vi "Keithley 2450 Read Multiple.vi"() -> ()   [LabVIEW 2024]
doc: "This example shows how to configure a measurement and take multiple readings."
uses:
  C:/Users/Public/OneDrive/Desktop/Keithley_2450_2470_1_4_0_LV2015_NewReadme2_2450-LV2015-1.4.0/Keithley 2450/Keithley 2450.lvlib
panel:
  in  "Compliance Level (0.1)":dbl=0.1
  in  "Output Level (0)":dbl
  in  "Source Mode  (0: Voltage)":u16(ring) items=["Voltage", "Current"]
  out "Resistance":sgl[](array[numeric])
  out "Current":sgl[](array[numeric])
  out "Voltage":sgl[](array[numeric])
  in  "VISA resource name":refnum<visa-resource-name>
  # "(c) 2021 National Instruments.  ALL RIGHTS RESERVED."
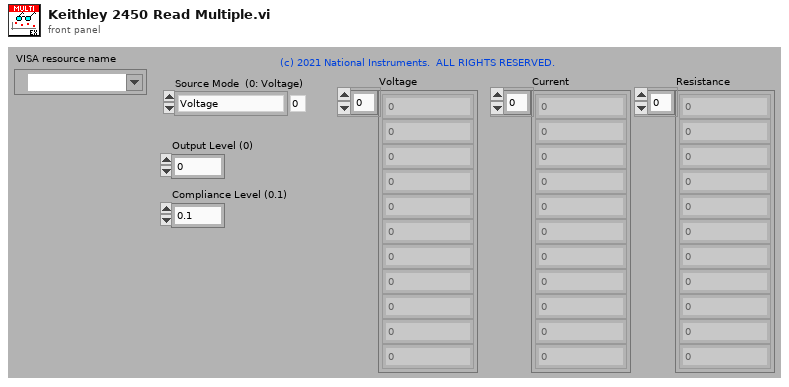
[diagram p1: front panel]
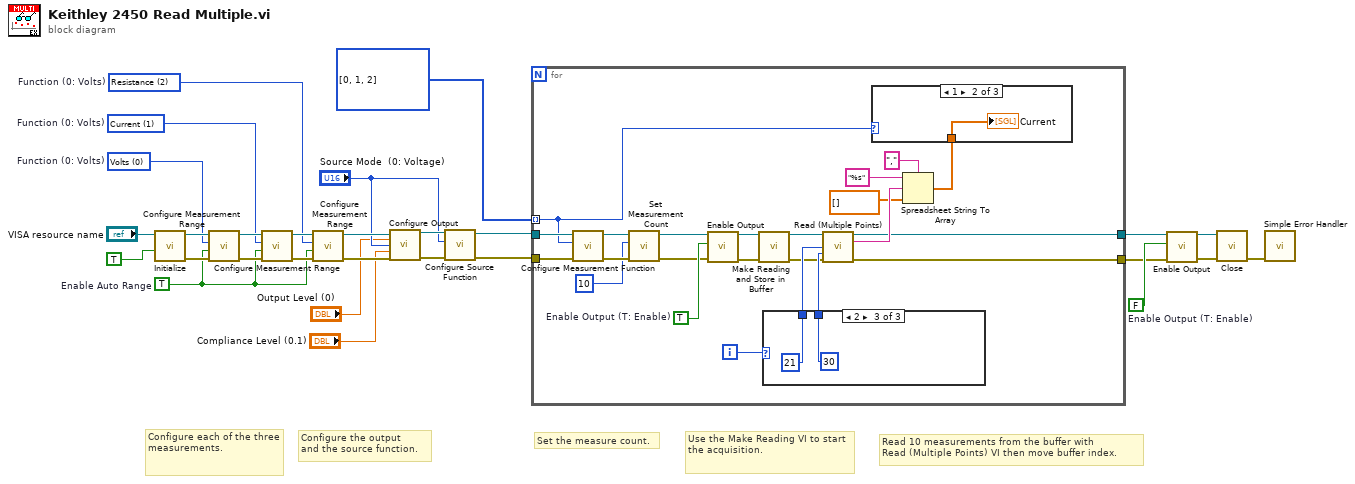
[diagram p0: block diagram]
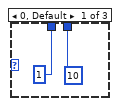
[diagram p2: hidden frame]
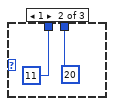
[diagram p3: hidden frame]
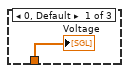
[diagram p4: hidden frame]
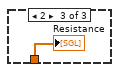
[diagram p5: hidden frame]
diagram:
  w9 = u16[] [0, 1, 2] items=["Volts", "Current", "Resistance"]
  w14 = FALSE  # Enable Output (T: Enable)
  w17 = u16 2 items=["Volts", "Current", "Resistance"]  # Function (0: Volts)
  w18 = u16 1 items=["Volts", "Current", "Resistance"]  # Function (0: Volts)
  w19 = u16 0 items=["Volts", "Current", "Resistance"]  # Function (0: Volts)
  w20 = TRUE  # Enable Auto Range
  # "Read 10 measurements from the buffer with \nRead (Multiple Points) VI then move buffer index."
  # "Set the measure count."
  # "Use the Make Reading VI to start the acquisition."
  # "Configure the output \nand the source function."
  # "Configure each of the three measurements."
  n1 = call "Initialize.vi"("Reset (True)"=TRUE, "VISA resource name"="VISA resource name") -> ("error out"=w25:errorcluster, "VISA resource name out"=w26:refnum<visa-resource-name>)  [unwired: 8 in]
  n2 = call "Configure Measurement Range.vi"("error in (no error)"=w25, "Enable Auto Range (T:Enable)"=w20, "Function (0: Volts)"=w19, "VISA resource name"=w26) -> ("error out"=w24:errorcluster, "VISA resource name out"=w23:refnum<visa-resource-name>)  [unwired: 6 in]
  n3 = call "Configure Measurement Range.vi"("error in (no error)"=w24, "Enable Auto Range (T:Enable)"=w20, "Function (0: Volts)"=w18, "VISA resource name"=w23) -> ("error out"=w21:errorcluster, "VISA resource name out"=w22:refnum<visa-resource-name>)  [unwired: 6 in]
  n4 = call "Configure Measurement Range.vi"("error in (no error)"=w21, "Enable Auto Range (T:Enable)"=w20, "Function (0: Volts)"=w17, "VISA resource name"=w22) -> ("error out"=w12:errorcluster, "VISA resource name out"=w13:refnum<visa-resource-name>)  [unwired: 6 in]
  n5 = call "Configure Output.vi"("VISA resource name"=w13, "Source Level (0)"="Output Level (0)", "Source Mode  (0: Voltage)"="Source Mode  (0: Voltage)", "Source Limit Level (0.1)"="Compliance Level (0.1)", "error in (no error)"=w12) -> ("VISA resource name out"=w7:refnum<visa-resource-name>, "error out"=w8:errorcluster)  [unwired: 9 in]
  n6 = call "Configure Source Function.vi"("error in (no error)"=w8, "Function (0: Volts)"="Source Mode  (0: Voltage)", "VISA resource name"=w7) -> ("error out"=w5:errorcluster, "VISA resource name out"=w6:refnum<visa-resource-name>)  [unwired: 7 in]
  n7 = for {
    tunnel: [w40] -> w11
    tunnel: [w39] -> w10
    tunnel: w5 -> [w51]
    tunnel: w6 -> [w50]
    tunnel: w9 -> [w49] mode=indexing
    i -> [w36]
    w33 = TRUE  # Enable Output (T: Enable)
    n8 = call "Configure Measurement Function.vi"("error in (no error)"=w51, "Function (0: Volts)"=w49, "VISA resource name"=w50) -> ("error out"=w48:errorcluster, "VISA resource name out"=w47:refnum<visa-resource-name>)  [unwired: 7 in]
    n9 = call "Set Measurement Count.vi"("error in (no error)"=w48, "Measurement Count"=u32 10 ("millisecond multiple"), "VISA resource name"=w47) -> ("error out"=w31:errorcluster, "VISA resource name out"=w32:refnum<visa-resource-name>)  [unwired: 7 in]
    n10 = call "Enable Output.vi"("error in (no error)"=w31, "Enable Output (T: Enable)"=w33, "VISA resource name"=w32) -> ("error out"=w29:errorcluster, "VISA resource name out"=w30:refnum<visa-resource-name>)  [unwired: 7 in]
    n11 = call "Make Reading and Store in Buffer.vi"("VISA resource name"=w30, "error in (no error)"=w29) -> ("VISA resource name out"=w35:refnum<visa-resource-name>, "error out"=w34:errorcluster)  [unwired: 12 in]
    n12 = case shown="2" w36 {
      tunnel: [u32 1 ("millisecond multiple") u32 11 ("millisecond multiple") u32 21 ("millisecond multiple")] -> w38
      tunnel: [u32 10 ("millisecond multiple") u32 20 ("millisecond multiple") u32 30 ("millisecond multiple")] -> w37
      frame 0, Default {
      }
      frame 1 {
      }
      frame 2 {
      }
    }
    n13 = call "Read (Multiple Points).vi"("VISA resource name"=w35, "Start Index (1)"=w38, "End Index (1)"=w37, "error in (no error)"=w34) -> ("VISA resource name out"=w40:refnum<visa-resource-name>, "Data out"=w45:string, "error out"=w39:errorcluster)  [unwired: 9 in]
    n14 = Spreadsheet String To Array(delimiter (Tab)=",", format string="%s", spreadsheet string=w45, array type (2D Dbl)=dbl[] []) -> (array=w44:dbl[])
    n15 = case shown="1" w49 {
      tunnel: w44 -> [w58 w59 w60]
      frame 0, Default {
        "Voltage" <- w58
      }
      frame 1 {
        "Current" <- w59
      }
      frame 2 {
        "Resistance" <- w60
      }
    }
  }
  n16 = call "Enable Output.vi"("error in (no error)"=w10, "Enable Output (T: Enable)"=w14, "VISA resource name"=w11) -> ("error out"=w15:errorcluster, "VISA resource name out"=w16:refnum<visa-resource-name>)  [unwired: 7 in]
  n17 = call "Close.vi"("error in (no error)"=w15, "VISA resource name"=w16) -> ("error out"=w28:errorcluster)  [unwired: 9 in]
  n18 = call <vilib>:"Simple Error Handler.vi"("error in (no error)"=w28) -> ()  [unwired: 4 in, 5 out]
